vi "main.vi"() -> ()   [LabVIEW 2014]
uses:
  States.ctl
  Read/Read Corvue/Read CorVue.lvclass
  Spectral Processing/Spectral Processing.lvclass
  Spectral Processing/Base Spectrum.vi
panel:
  out "Current State":T1
  in  "Depth":u32=50
  in  "Window Width":u32=10
  in  "Show BScan":bool
  in  "BPF Spectrum":bool
  in  "Base Spectrum":bool
  in  "A-Scan":u32(slide) scale=-1.0..667.0
  in  "Stop Button":bool
  in  "B-Scan":u32(slide) scale=0.0..300.0
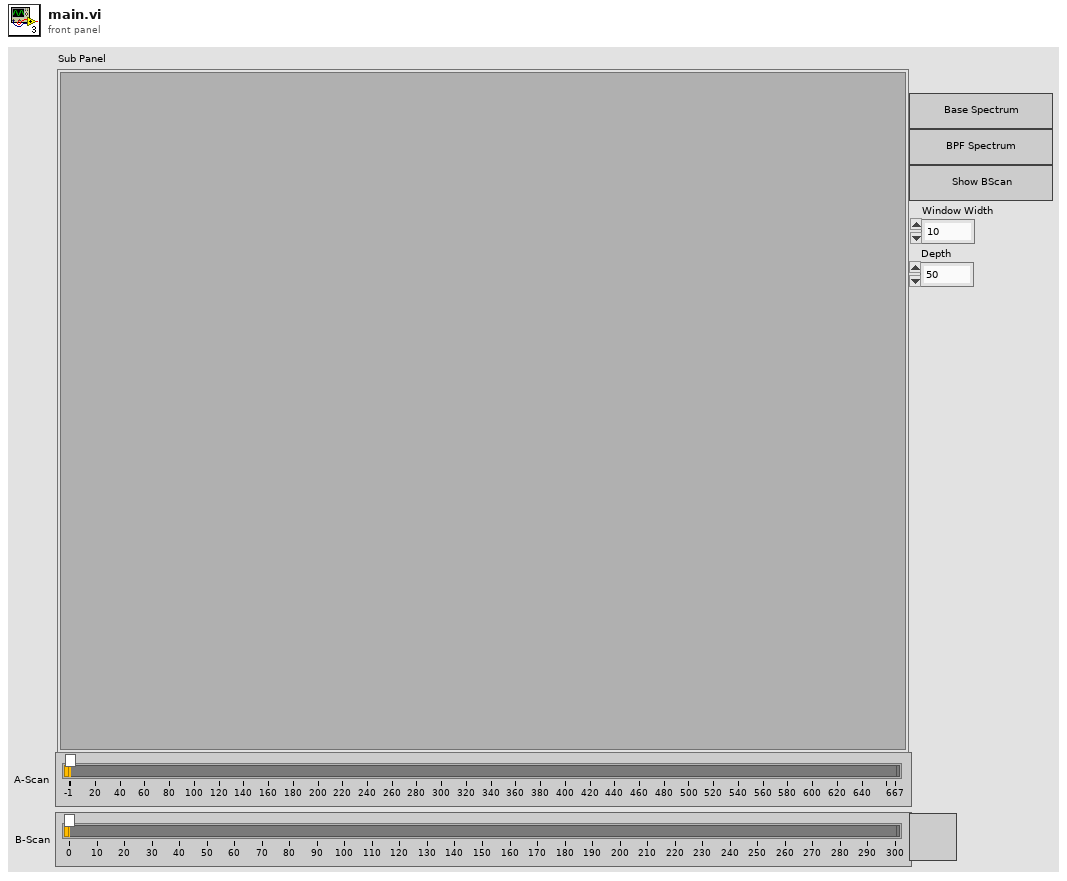
[diagram p1: front panel]
types:
  T1 = typedef "States.ctl" = enum16{"Open", "Close", "Process", "Read", "Compute BScan", "BPF Spectrum"}
  T2 = typedef "Read.lvclass/BScan.ctl" = cluster{"Points Per A-Scan":dbl, "A-Scans per B-Scan":dbl}
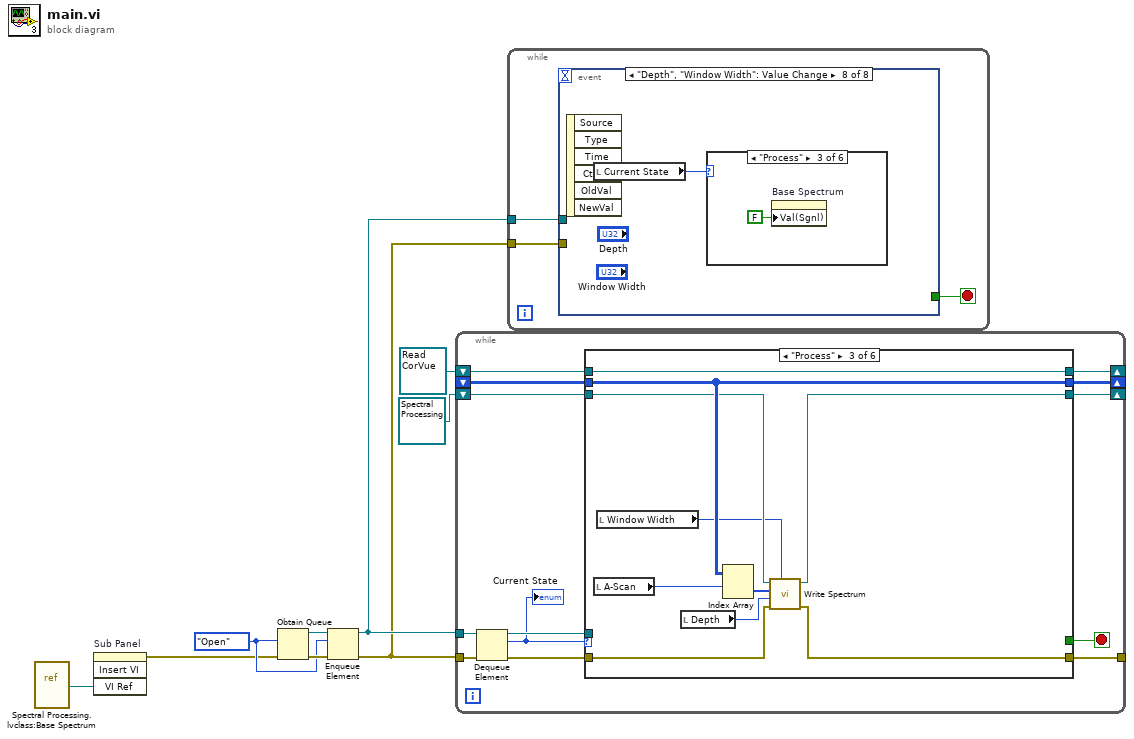
[diagram p0: block diagram]
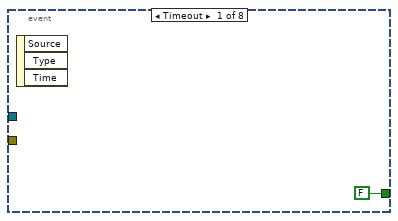
[diagram p2: hidden frame]
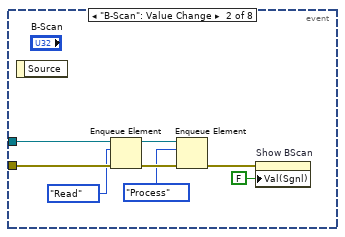
[diagram p3: hidden frame]
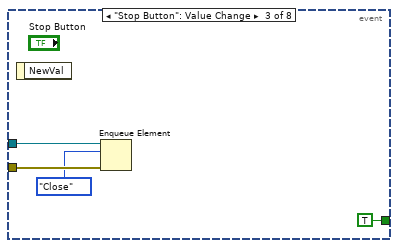
[diagram p4: hidden frame]
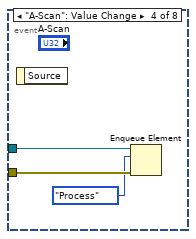
[diagram p5: hidden frame]
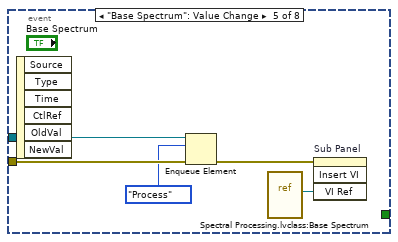
[diagram p6: hidden frame]
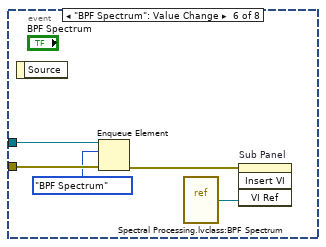
[diagram p7: hidden frame]
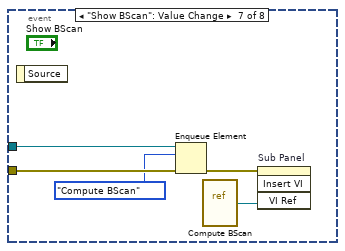
[diagram p8: hidden frame]
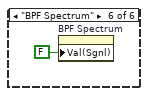
[diagram p13: hidden frame]
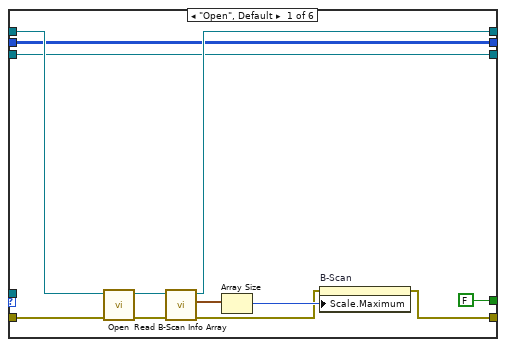
[diagram p14: hidden frame]
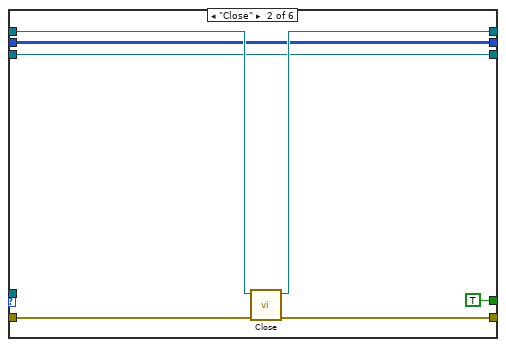
[diagram p15: hidden frame]
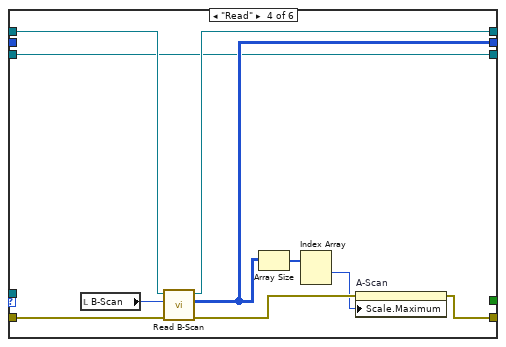
[diagram p16: hidden frame]
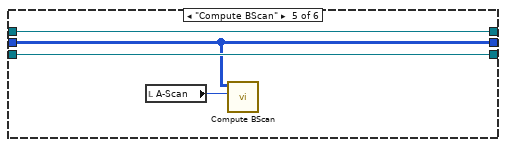
[diagram p17: hidden frame]
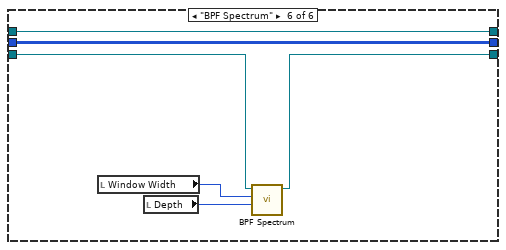
[diagram p18: hidden frame]
diagram:
  w6 = States."Open"
  n1 = vi-ref "Spectral Processing.lvclass:Base Spectrum.vi"() -> (w1:refnum<vi>)
  n2 = invoke on="Sub Panel" class="SubPanel" method="Insert VI"("VI Ref"=w1) -> (error out=w2:errorcluster)  [unwired: 3 in, 3 out]
  n3 = Obtain Queue(element data type=w6, error in (no error)=w2) -> (queue out=w8:refnum<queue>, error out=w7:errorcluster)  [unwired: 3 in, 1 out]
  n4 = Enqueue Element(queue=w8, element=w6, error in (no error)=w7) -> (queue out=w5:refnum<queue>, error out=w4:errorcluster)  [unwired: 1 in, 1 out]
  n5 = while {
    shift-right: [w17] -> _
    shift-left: refnum<class "Read CorVue.lvclass"> refnum ("Read CorVue.lvclass") -> [w20]
    tunnel: w4 -> [w22]
    tunnel: w5 -> [w21]
    tunnel: [w16] -> _
    shift-right: [w14] -> _
    shift-left: _ -> [w13]
    shift-right: [w11] -> _
    shift-left: refnum<class "Spectral Processing.lvclass"> refnum ("Spectral Processing.lvclass") -> [w12]
    stop <- w15 stop-if-true
    n6 = Dequeue Element(queue=w21, error in (no error)=w22) -> (queue out=w18:refnum<queue>, element=w10:T1, error out=w19:errorcluster)  [unwired: 1 in, 1 out]
    "Current State" <- w10
    n7 = case shown="\"Process\"" w10 {
      tunnel: w20 -> [w33 w40 w51 w60 w64 w71]
      tunnel: w19 -> [w34 w41 w45 w61 _ _]
      tunnel: w18 -> [_ _ _ _ _ _]
      tunnel: [w29 w39 w51 w59 w64 w71] -> w17
      tunnel: [w25 w38 w44 w56 _ _] -> w16
      tunnel: [FALSE TRUE _ _ _ _] -> w15
      tunnel: [w24 w36 w49 w54 w63 w70] -> w14
      tunnel: w13 -> [w24 w36 w49 _ w63 w70]
      tunnel: w12 -> [w23 w35 w47 w52 w65 w69]
      tunnel: [w23 w35 w46 w52 w65 w68] -> w11
      frame "Open", Default {
        n8 = call-dynamic "Open.vi"("error in (no error)"=w34, "Read CorVue in"=w33) -> ("error out"=w30:errorcluster, "Read CorVue out"=w31:refnum<class "Read CorVue.lvclass">)  [unwired: 8 in]
        n9 = call-dynamic "Read B-Scan Info Array.vi"("error in (no error)"=w30, "Read in"=w31) -> ("error out"=w26:errorcluster, "B-Scan Info Array"=w28:T2[], "Read out"=w29:refnum<class "Read CorVue.lvclass">)  [unwired: 7 in]
        n10 = Array Size(array=w28) -> (size(s)=w27:i32)
        n11 = property on="B-Scan" class="Slide (strict)"(error in=w26, "Scale.Maximum"=w27) -> (error out=w25:errorcluster)  [unwired: 1 in, 1 out]
      }
      frame "Close" {
        n12 = call-dynamic "Close.vi"("error in (no error)"=w41, "Read in"=w40) -> ("error out"=w38:errorcluster, "Read out"=w39:refnum<class "Read CorVue.lvclass">)  [unwired: 8 in]
      }
      frame "Process" {
        n13 = local read "A-Scan"() -> (w50:u32)
        n14 = local read "Window Width"() -> (w42:u32)
        n15 = local read "Depth"() -> (w43:u32)
        n16 = Index Array(array=w49, index (row)=w50) -> (element=w48:u16[])  [unwired: 1 in]
        n17 = call-dynamic "Write Spectrum.vi"("Window Width"=w42, "error in (no error)"=w45, "Depth"=w43, "Spectrum"=w48, "Spectral Processing in"=w47) -> ("error out"=w44:errorcluster, "Spectral Processing out"=w46:refnum<class "Spectral Processing.lvclass">)  [unwired: 5 in]
      }
      frame "Read" {
        n18 = local read "B-Scan"() -> (w58:u32)
        n19 = call-dynamic "Read B-Scan.vi"("error in (no error)"=w61, "Index"=w58, "Read in"=w60) -> ("error out"=w57:errorcluster, "Raw B-Scan"=w54:u16[][], "Read out"=w59:refnum<class "Read CorVue.lvclass">)  [unwired: 6 in]
        n20 = Array Size(array=w54) -> (size(s)=w55:i32[])
        n21 = Index Array(array=w55) -> (element #1=w53:i32)  [unwired: 2 in, 1 out]
        n22 = property on="A-Scan" class="Slide (strict)"(error in=w57, "Scale.Maximum"=w53) -> (error out=w56:errorcluster)  [unwired: 1 in, 1 out]
      }
      frame "Compute BScan" {
        n23 = local read "A-Scan"() -> (w62:u32)
        n24 = call "Compute BScan.vi"("A-Scan"=w62, "Array"=w63) -> ()  [unwired: 10 in]
      }
      frame "BPF Spectrum" {
        n25 = local read "Window Width"() -> (w66:u32)
        n26 = local read "Depth"() -> (w67:u32)
        n27 = call-dynamic "BPF Spectrum.vi"("Depth"=w67, "Window Width"=w66, "Spectral Processing in"=w69) -> ("Spectral Processing out"=w68:refnum<class "Spectral Processing.lvclass">)  [unwired: 7 in, 1 out]
      }
    }
  }
  n28 = while {
    tunnel: w5 -> [w73]
    tunnel: w4 -> [w72]
    stop <- w74 stop-if-true
    n29 = event shown="[7] \"Depth\", \"Window Width\": Value Change" {
      selector: _ -> [_ _ _ _ _ _ _ _]
      dyn-events: _ -> [_ _ _ _ _ _ _ _]
      timeout: _ -> [_ _ _ _ _ _ _ _]
      tunnel: [FALSE _ TRUE _ _ _ _ _] -> w74
      tunnel: w73 -> [_ w83 w86 w90 w94 w100 w105 _]
      tunnel: w72 -> [_ w82 w85 w89 w93 w99 w104 _]
      event Timeout {
        n30 = event-data() -> ()  [unwired: 1 in, 3 out]
      }
      event "B-Scan": Value Change {
        n31 = event-data() -> ()  [unwired: 1 in, 1 out]
        n32 = Enqueue Element(queue=w83, element=States."Read", error in (no error)=w82) -> (queue out=w79:refnum<queue>, error out=w80:errorcluster)  [unwired: 1 in, 1 out]
        n33 = Enqueue Element(queue=w79, element=States."Process", error in (no error)=w80) -> (error out=w77:errorcluster)  [unwired: 1 in, 2 out]
        n34 = property on="Show BScan" class="Bool (strict)"(error in=w77, "Val(Sgnl)"=FALSE ("Value (Signaling)")) -> ()  [unwired: 1 in, 2 out]
      }
      event "Stop Button": Value Change {
        n35 = event-data() -> ()  [unwired: 1 in, 1 out]
        n36 = Enqueue Element(queue=w86, element=States."Close", error in (no error)=w85) -> ()  [unwired: 1 in, 3 out]
      }
      event "A-Scan": Value Change {
        n37 = event-data() -> ()  [unwired: 1 in, 1 out]
        n38 = Enqueue Element(queue=w90, element=States."Process", error in (no error)=w89) -> ()  [unwired: 1 in, 3 out]
      }
      event "Base Spectrum": Value Change {
        n39 = event-data() -> ()  [unwired: 1 in, 6 out]
        n40 = Enqueue Element(queue=w94, element=States."Process", error in (no error)=w93) -> (error out=w91:errorcluster)  [unwired: 1 in, 2 out]
        n41 = vi-ref "Spectral Processing.lvclass:Base Spectrum.vi"() -> (w95:refnum<vi>)
        n42 = invoke on="Sub Panel" class="SubPanel" method="Insert VI"(error in=w91, "VI Ref"=w95) -> ()  [unwired: 2 in, 4 out]
      }
      event "BPF Spectrum": Value Change {
        n43 = event-data() -> ()  [unwired: 1 in, 1 out]
        n44 = Enqueue Element(queue=w100, element=States."BPF Spectrum", error in (no error)=w99) -> (error out=w96:errorcluster)  [unwired: 1 in, 2 out]
        n45 = vi-ref "Spectral Processing.lvclass:BPF Spectrum.vi"() -> (w97:refnum<vi>)
        n46 = invoke on="Sub Panel" class="SubPanel" method="Insert VI"(error in=w96, "VI Ref"=w97) -> ()  [unwired: 2 in, 4 out]
      }
      event "Show BScan": Value Change {
        n47 = event-data() -> ()  [unwired: 1 in, 1 out]
        n48 = Enqueue Element(queue=w105, element=States."Compute BScan", error in (no error)=w104) -> (error out=w102:errorcluster)  [unwired: 1 in, 2 out]
        n49 = vi-ref "Compute BScan.vi"() -> (w101:refnum<vi>)
        n50 = invoke on="Sub Panel" class="SubPanel" method="Insert VI"(error in=w102, "VI Ref"=w101) -> ()  [unwired: 2 in, 4 out]
      }
      event "Depth", "Window Width": Value Change {
        n51 = event-data() -> ()  [unwired: 1 in, 6 out]
        n52 = local read "Current State"() -> (w106:T1)
        n53 = case shown="\"Process\"" w106 {
          frame "Open", Default {
          }
          frame "Close" {
          }
          frame "Process" {
            n54 = property on="Base Spectrum" class="Bool (strict)"("Val(Sgnl)"=FALSE ("Value (Signaling)")) -> ()  [unwired: 2 in, 2 out]
          }
          frame "Read" {
          }
          frame "Compute BScan" {
          }
          frame "BPF Spectrum" {
            n55 = property on="BPF Spectrum" class="Bool (strict)"("Val(Sgnl)"=FALSE ("Value (Signaling)")) -> ()  [unwired: 2 in, 2 out]
          }
        }
      }
    }
  }
